vi "Process.vi"() -> ()   [LabVIEW 2020, in "Test Actor.lvclass"]
uses:
  Test Actor.lvclass
  Base Actor/Actor/Actor.lvclass/Actor.ctl
  Base Actor/Sequencer/Sequencer.lvclass/Sequencer.ctl
  Test Actor.lvclass/Test Actor.ctl
  Count Behaviour.ctl
  <vilib>/Utility/High Resolution Relative Seconds.vi
  C:/dev/PGS/2001 - TBCM/Source/RT/RTAF/Source/RTAF/Actors/Base Actor/Actor/Actor.lvclass
  Base Actor/Actor/Actor.lvclass
panel:
  out "Iteration":i32
  in  "Tick Period [ms]":i32=5 min=2 step=1
  out "Tick Period [s]":dbl format="%.1p"
  out "Numeric":i32
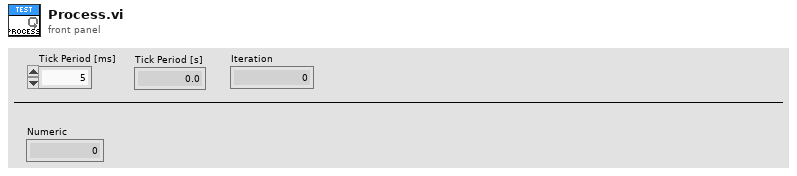
[diagram p1: front panel]
types:
  T1 = enum32{"Invalid", "Standard", "Closed", "Hidden", "Minimized", "Maximized"}
  T2 = typedef "Test Actor.lvclass/Count Behaviour.ctl" = enum16{"Stopped", "Up", "Down"}
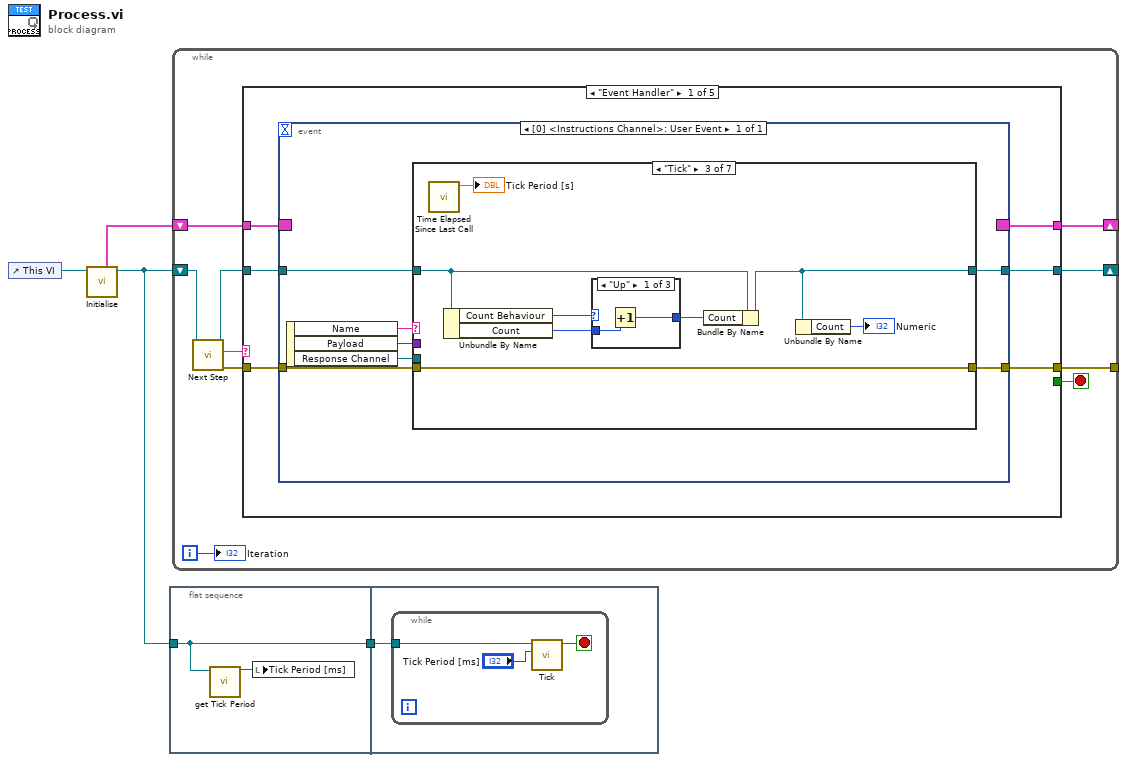
[diagram p0: block diagram]
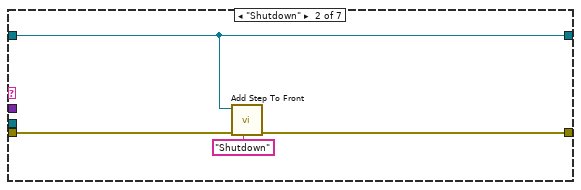
[diagram p3: hidden frame]
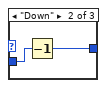
[diagram p4: hidden frame]
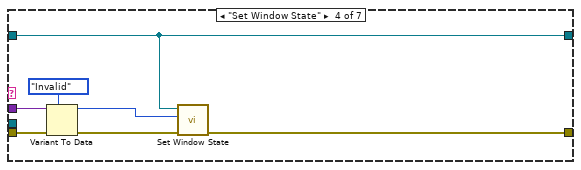
[diagram p6: hidden frame]
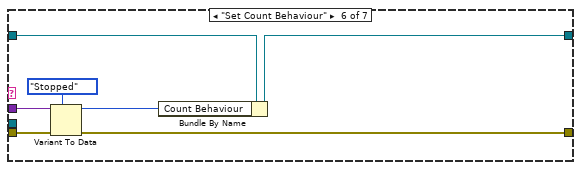
[diagram p8: hidden frame]
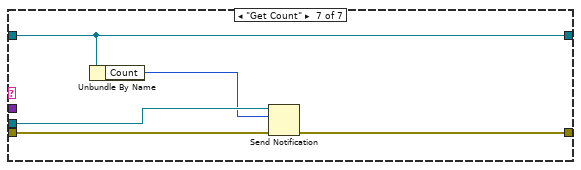
[diagram p9: hidden frame]
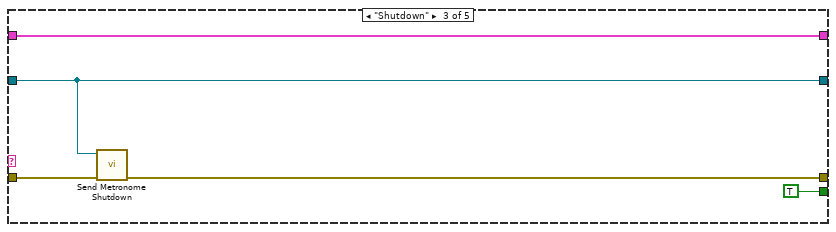
[diagram p11: hidden frame]
diagram:
  n1 = control-ref of="This VI"() -> (w3:refnum<vi>)
  n2 = call "Initialise.vi"("Process"=w3) -> ("Actor out"=w1:refnum<class "Test Actor.lvclass">, "Mailboxes"=w2:cluster{"Mailbox":refnum<event-registration>})  [unwired: 8 in, 1 out]
  n3 = flat-sequence {
    tunnel: w1 -> [w6]
    tunnel: [w6] -> w4
    tunnel: w4 -> [w7]
    frame #0 {
      n4 = call "get Tick Period.vi"("Actor in"=w6) -> ("Tick Period [ms]"=w5:i32)  [unwired: 10 in]
      n5 = local write "Tick Period [ms]"(w5) -> ()
    }
    frame #1 {
      n6 = while {
        tunnel: w7 -> [w10]
        stop <- w8 stop-if-true
        n7 = call "Tick.vi"("Tick Period [ms]"="Tick Period [ms]", "Actor in"=w10) -> ("Shutdown"=w8:bool)  [unwired: 9 in]
      }
    }
  }
  n8 = while {
    shift-right: [w19] -> _
    shift-left: w1 -> [w16]
    tunnel: [w18] -> _
    shift-right: [w11] -> _
    shift-left: w2 -> [w20]
    i -> [w12]
    stop <- w13 stop-if-true
    n9 = call "Next Step.vi"("Actor in"=w16) -> ("error out"=w17:errorcluster, "Next Step"=w14:string, "Actor out"=w15:refnum<class "Test Actor.lvclass">)  [unwired: 8 in]
    n10 = case shown="\"Event Handler\"" w14 {
      tunnel: w20 -> [w21 w73 w76 w81 w84]
      tunnel: [_ _ TRUE _ _] -> w13
      tunnel: w15 -> [w26 w75 w79 w83 w86]
      tunnel: [w25 w75 w79 w83 w86] -> w19
      tunnel: [w24 w74 w78 w82 w85] -> w18
      tunnel: w17 -> [w23 w74 w77 w82 w85]
      tunnel: [w22 w73 w76 w81 w84] -> w11
      frame "Event Handler" {
        n11 = event shown="[0] <Instructions Channel>: User Event" {
          selector: w21 -> [_]
          dyn-events: [_] -> w22
          timeout: _ -> [_]
          tunnel: w26 -> [w31]
          tunnel: [w30] -> w25
          tunnel: [w28] -> w24
          tunnel: w23 -> [w27]
          event User Event {
            n12 = event-data() -> ("Name"=w33:string, "Payload"=w32:variant, "Response Channel"=w29:refnum<notifier>)  [unwired: 1 in]
            n13 = case shown="\"Tick\"" w33 {
              tunnel: w32 -> [_ _ _ w58 _ w65 _]
              tunnel: w31 -> [w34 w38 w42 w54 w60 w66 w72]
              tunnel: [w34 w38 w41 w54 w60 w67 w72] -> w30
              tunnel: w29 -> [_ _ _ _ _ _ w71]
              tunnel: [_ w37 w40 w55 w59 w62 w68] -> w28
              tunnel: w27 -> [_ w36 w40 w57 w59 w61 w69]
              frame Default {
              }
              frame "Shutdown" {
                n14 = call "Add Step To Front.vi"("Step Name"="Shutdown", "error in (no error)"=w36, "Actor in"=w38) -> ("error out"=w37:errorcluster)  [unwired: 8 in]
              }
              frame "Tick" {
                n15 = call "Time Elapsed Since Last Call.vi"() -> ("Time Elapsed Since Last Call [s]"=→"Tick Period [s]":dbl)  [unwired: 11 in]
                n16 = Unbundle By Name(w42) -> ("Count Behaviour"=w43:T2, "Count"=w46:i32)
                n17 = case shown="\"Up\"" w43 {
                  tunnel: w46 -> [w48 w50 w51]
                  tunnel: [w47 w49 w51] -> w45
                  frame "Up" {
                    n18 = Increment(x=w48) -> (x+1=w47:i32)
                  }
                  frame "Down" {
                    n19 = Decrement(x=w50) -> (x-1=w49:i32)
                  }
                  frame "Stopped" {
                  }
                }
                n20 = Bundle By Name(cluster=w42, "Count"=w45) -> (w41:refnum<class "Test Actor.lvclass">)
                n21 = Unbundle By Name(w41) -> ("Count"=→"Numeric":i32)
              }
              frame "Set Window State" {
                n22 = Variant To Data(error in=w57, type=T1."Invalid", Variant=w58) -> (data=w53:T1, error out=w56:errorcluster)
                n23 = call "Set Window State.vi"("error in (no error)"=w56, "State"=w53, "Actor in"=w54) -> ("error out"=w55:errorcluster)  [unwired: 8 in]
              }
              frame "----------------------------------" {
              }
              frame "Set Count Behaviour" {
                n24 = Variant To Data(error in=w61, type=Count_Behaviour."Stopped" ("Count Behaviour"), Variant=w65) -> (data=w63:T2, error out=w62:errorcluster)
                n25 = Bundle By Name(cluster=w66, "Count Behaviour"=w63) -> (w67:refnum<class "Test Actor.lvclass">)
              }
              frame "Get Count" {
                n26 = Unbundle By Name(w72) -> ("Count"=w70:i32)
                n27 = Send Notification(notification=w70, notifier=w71, error in (no error)=w69) -> (error out=w68:errorcluster)  [unwired: 1 out]
              }
            }
          }
        }
      }
      frame "Error Handler" {
      }
      frame "Shutdown" {
        n28 = call "Send Metronome Shutdown.vi"("error in (no error)"=w77, "Actor in"=w79) -> ("error out"=w78:errorcluster)  [unwired: 9 in]
      }
      frame "Unhandled Step", Default {
      }
      frame "-----------------------------------" {
      }
    }
    "Iteration" <- w12
  }
